vi "Destroy.vi"(8 "error in (no error)":errorcluster, 11 "reference in":refnum<class "RemoteControl.lvclass">) -> (0 "error out":errorcluster, 3 "reference out":refnum<class "RemoteControl.lvclass">)   [LabVIEW 2020, in "RemoteControl.lvclass"]
uses:
  RemoteControl.lvclass
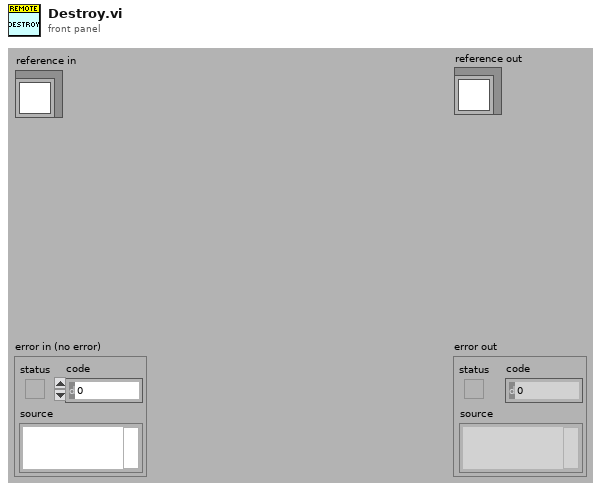
[diagram p1: front panel]
types:
  T1 = typedef "RemoteControl.lvclass/ObjectAttributes.ctl" = cluster{"OnCommands":refnum<class "Command.lvclass">[], "OffCommands":refnum<class "Command.lvclass">[], "UndoCommand":refnum<class "Command.lvclass">}
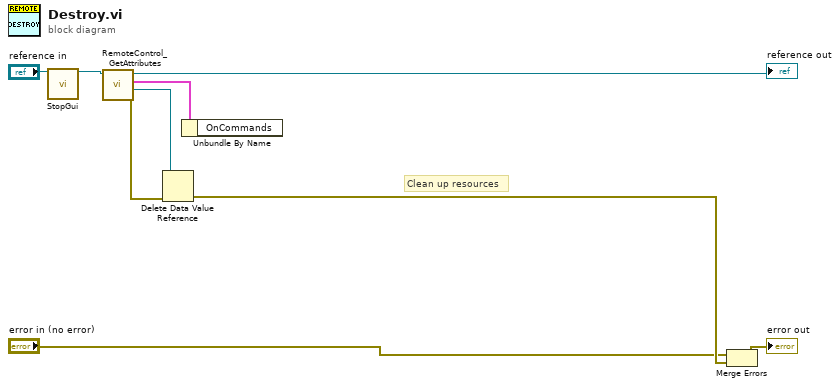
[diagram p0: block diagram]
diagram:
  # "Clean up resources"
  n1 = call "StopGui.vi"("reference in"="reference in") -> ("reference out"=w1:refnum<class "RemoteControl.lvclass">)  [unwired: 17 in, 1 out]
  n2 = call "RemoteControl_GetAttributes.vi"("reference in"=w1) -> ("error out"=w7:errorcluster, "DataRef"=w6:refnum<data-value>, "Data"=w5:T1, "reference out"=→"reference out":refnum<class "RemoteControl.lvclass">)  [unwired: 7 in]
  n3 = Delete Data Value Reference(data value reference=w6, error in=w7) -> (error out=w4:errorcluster)  [unwired: 1 out]
  n4 = Unbundle By Name(w5) -> ()  [unwired: 1 out]
  n5 = Merge Errors("error in (no error)", w4) -> (→"error out":errorcluster)
